vi "Decode BiDirectional Tag (Erroneous Type).vi"(8 "error in (no error)":errorcluster, 11 "PicoQuant Tag":T1 {"TagType" format="%.0x"}) -> (0 "error out":errorcluster, 3 "Bidirectional":bool)   [LabVIEW 2021, in "PTU Files.lvlib"]
uses:
  PTU Files.lvlib
  PicoQuant Header Tag.ctl
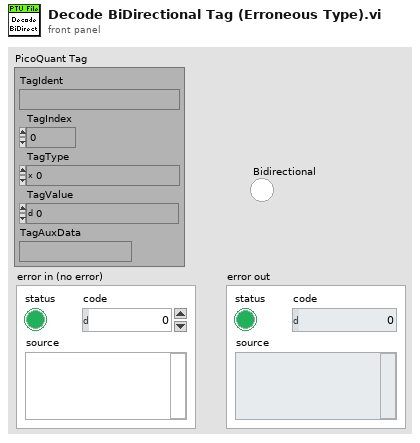
[diagram p1: front panel]
types:
  T1 = typedef "PTU Files.lvlib/PicoQuant Header Tag.ctl" = cluster{"TagIdent":string, "TagIndex":i32, "TagType":i32, "TagValue":i64, "TagAuxData":string}
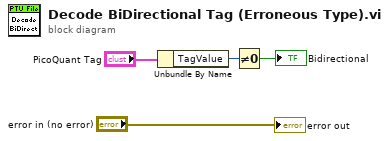
[diagram p0: block diagram]
diagram:
  n1 = Unbundle By Name("PicoQuant Tag") -> ("TagValue"=w2:i64)
  n2 = Not Equal To 0?(x=w2) -> (x != 0?=→"Bidirectional":bool)
  "error out" <- "error in (no error)"
